vi "SPI Write & Read.vi"(8 "error in (no error)":errorcluster, 10 "Data":u8[](array[numeric]), 11 "LINX SPI in":refnum<class "LINX SPI.lvclass">) -> (0 "error out":errorcluster, 2 "Read Data":u8[](array[numeric]), 3 "LINX SPI out":refnum<class "LINX SPI.lvclass">)   [LabVIEW 2020, in "LINX SPI.lvclass"]
uses:
  LINX SPI.lvclass
  LINX SPI.lvclass/LINX SPI.ctl
  Read LINX Resource.vi
  Read CS Configuration.vi
  Write LINX Resource.vi
  <vilib>/MakerHub/LINX/Private/Local IO/LinxSpiWriteRead.vi
  <vilib>/MakerHub/LINX/Public/Utilities/Check Channel.vi
  <vilib>/MakerHub/LINX/Private/Local IO/Handle Errors.vi
  <vilib>/MakerHub/LINX/Private/Utilties/Generate Error.vi
  <vilib>/MakerHub/LINX/LMH-LINX.lvlib
  <vilib>/MakerHub/LINX/Public/Peripherals/SPI/SPI Write Read 1 Frame.vi
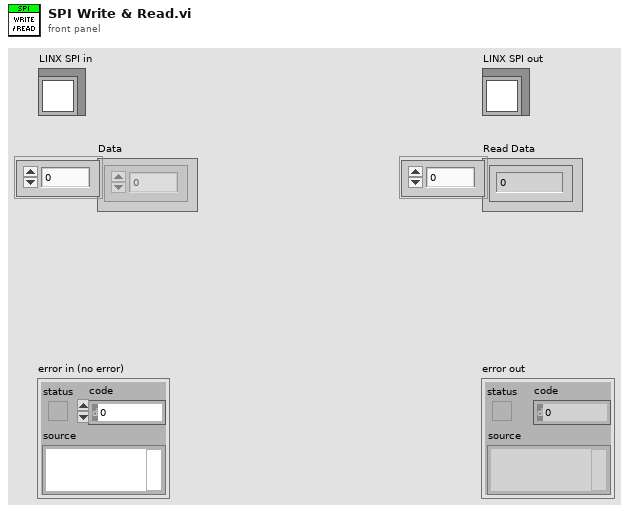
[diagram p1: front panel]
types:
  T1 = typedef "LMH-LINX.lvlib/LINX Ref.ctl" = cluster{"IO":T2, "Interface":T3, "LINX Device Config":T4}
  T2 = typedef "LMH-LINX.lvlib/Platform.ctl" = enum16{"Remote", "Local"}
  T3 = typedef "LMH-LINX.lvlib/Interface.ctl" = enum16{"Serial", "TCP"}
  T4 = typedef "LMH-LINX.lvlib/Device.lvlib/LINX Device Config.ctl" = cluster{"Interface":T3, "COM Port":refnum<visa-resource-name>, "TCP Configuration":T5, "Device Family":u8, "Device ID":u8, "Device Name":string, "TCP Ref":refnum<k5>, "Channels":T6}
  T5 = typedef "LMH-LINX.lvlib/Device.lvlib/TCP Config.ctl" = cluster{"IP Address":string, "Port":u16}
  T6 = typedef "LMH-LINX.lvlib/Channels.ctl" = cluster{"DI":u8[], "DO":u8[], "AI":u8[], "AO":u8[], "PWM":u8[], "QE":u8[], "UART":u8[], "I2C 2":u8[], "SPI":u8[], "CAN":u8[], "Servo":u8[], "AI Ref (V)":dbl, "AI Resolution (Bits)":u8, "AO Ref (V)":dbl, "AO Resolution (Bits)":u8}
  T7 = typedef "LMH-LINX.lvlib/SPI CS Config.ctl" = cluster{"CS Channel":u8, "CS Logic Level":T8}
  T8 = typedef "LMH-LINX.lvlib/SPI CS Logic Level.ctl" = enum8{"Active Low", "Active High"}
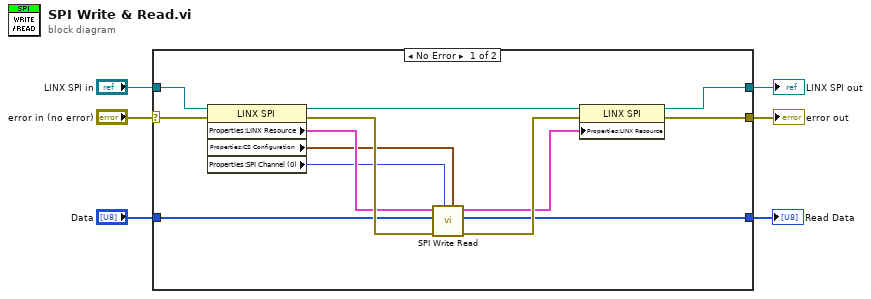
[diagram p0: block diagram]
diagram:
  n1 = case shown="No Error" "error in (no error)" {
    selector: "error in (no error)" -> [w18 w21]
    tunnel: [w13 w21] -> w5
    tunnel: [w12 w20] -> w3
    tunnel: "LINX SPI in" -> [w19 w20]
    tunnel: [w9 _] -> w2
    tunnel: "Data" -> [w8 _]
    frame No Error {
      n2 = property class="LINX SPI"(reference=w19, error in=w18) -> (reference out=w16:refnum<class "LINX SPI.lvclass">, error out=w17:errorcluster, "Properties:LINX Resource"=w14:T1, "Properties:CS Configuration"=w10:T7, "Properties:SPI Channel (0)"=w7:u8)
      n3 = call-poly <vilib>:"SPI Write Read.vi"("CS Configuration"=w10, "SPI Channel (0)"=w7, "Error In"=w17, "Data"=w8, "LINX Resource"=w14) -> ("Error Out"=w15:errorcluster, "Read Data"=w9:u8[], "LINX Resource"=w11:T1)  [unwired: 3 in, 1 out]
      n4 = property class="LINX SPI"(reference=w16, error in=w15, "Properties:LINX Resource"=w11) -> (reference out=w12:refnum<class "LINX SPI.lvclass">, error out=w13:errorcluster)
    }
    frame Error {
    }
  }
  "error out" <- w5
  "LINX SPI out" <- w3
  "Read Data" <- w2
